vi "Blink LEDArray Control.vi"(6 "Update Interval(1000 ms)":u32=1000, 7 "LED Array":refnum<vi>, 8 "error in (no error)":errorcluster, 11 "Enable":bool) -> (0 "error out":errorcluster)   [LabVIEW 2017]
doc: "Makes the boolean array behind an LED array control blink, rotating the array by one position every interval (ms). Wire Enable to start and stop the blinking."
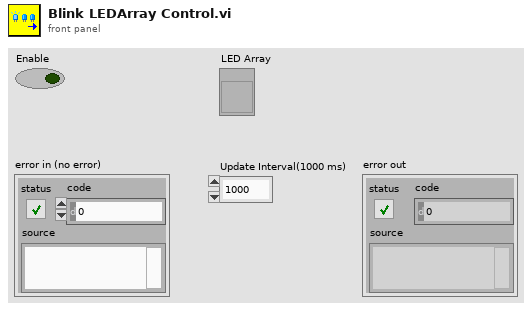
[diagram p1: front panel]
types:
  T1 = typedef "Def-3LEDs.ctl" = bool[]
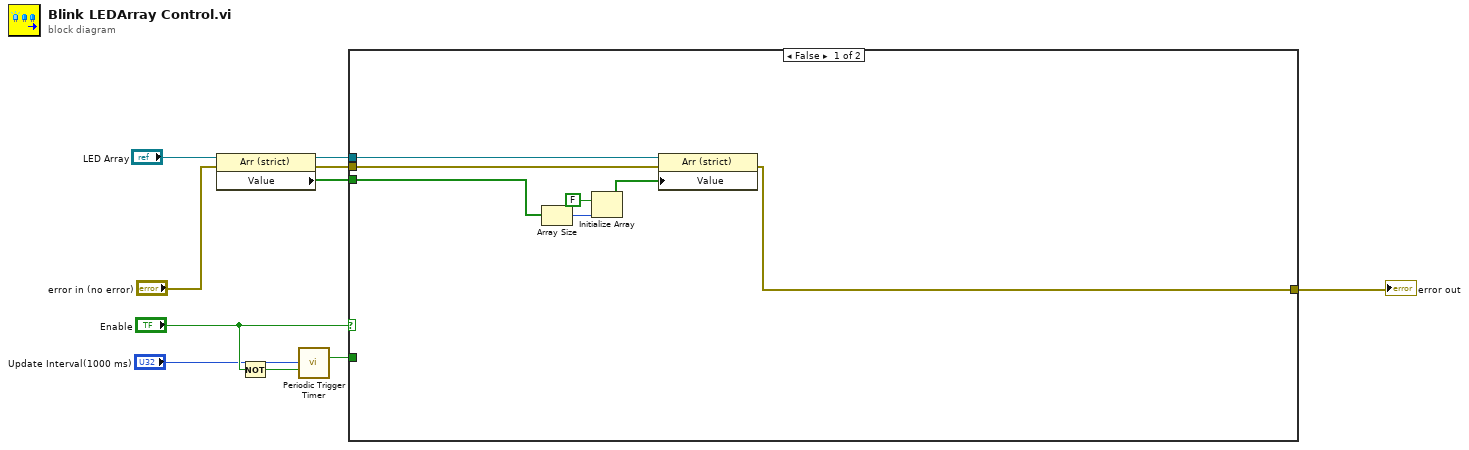
[diagram p0: block diagram]
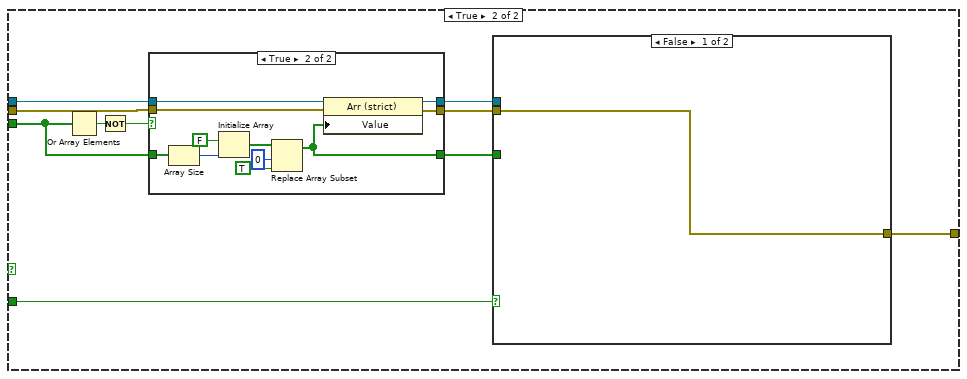
[diagram p2: hidden frame]
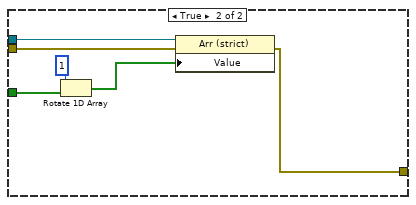
[diagram p4: hidden frame]
diagram:
  n1 = property on="Property Node" class="Arr (strict)"(reference="LED Array", error in="error in (no error)") -> (reference out=w1:refnum<vi>, error out=w8:errorcluster, "Value"=w2:T1)
  n2 = Not(x="Enable") -> (.not. x?=w7:bool)
  n3 = call "Periodic Trigger Timer.vi"("time (ms)"="Update Interval(1000 ms)", "reset"=w7) -> ("Triggered"=w5:bool)  [unwired: 11 in, 2 out]
  n4 = case shown="False" "Enable" {
    tunnel: w1 -> [w17 w25]
    tunnel: w2 -> [w16 w22]
    tunnel: w5 -> [_ w27]
    tunnel: w8 -> [w12 w18]
    tunnel: [w11 w21] -> w10
    frame False {
      n5 = Array Size(array=w16) -> (size(s)=w15:i32)
      n6 = Initialize Array(FALSE ("液压卸荷指示灯2"), w15) -> (w13:bool[])
      n7 = property class="Arr (strict)"(reference=w17, error in=w12, "Value"=w13) -> (error out=w11:errorcluster)  [unwired: 1 out]
    }
    frame True {
      n8 = Or Array Elements(Boolean array=w22) -> (logical OR=w24:bool)
      n9 = Not(x=w24) -> (.not. x?=w23:bool)
      n10 = case shown="True" w23 {
        tunnel: [w30 w41] -> w26
        tunnel: w25 -> [w30 w40]
        tunnel: w22 -> [w29 w37]
        tunnel: [w29 w33] -> w20
        tunnel: [w28 w32] -> w19
        tunnel: w18 -> [w28 w31]
        frame False {
        }
        frame True {
          n11 = Array Size(array=w37) -> (size(s)=w39:i32)
          n12 = Initialize Array(FALSE ("液压卸荷指示灯2"), w39) -> (w36:bool[])
          n13 = Replace Array Subset(array=w36, new element=TRUE ("液压卸荷指示灯2"), index=0) -> (w33:bool[])
          n14 = property class="Arr (strict)"(reference=w40, error in=w31, "Value"=w33) -> (reference out=w41:refnum<vi>, error out=w32:errorcluster)
        }
      }
      n15 = case shown="False" w27 {
        tunnel: w26 -> [_ w48]
        tunnel: w20 -> [_ w47]
        tunnel: [w42 w44] -> w21
        tunnel: w19 -> [w42 w43]
        frame False {
        }
        frame True {
          n16 = Rotate 1D Array(1:w47, 2:1 ("n")) -> (0:w45:T1)
          n17 = property class="Arr (strict)"(reference=w48, error in=w43, "Value"=w45) -> (error out=w44:errorcluster)  [unwired: 1 out]
        }
      }
    }
  }
  "error out" <- w10
